vi "Parse (Write To EEPROM).vi"(7 "Message In":string) -> (8 "Word Sent To EEPROM":sgl)   [LabVIEW 2012, in "MicroStrain 3DM-GXx.lvlib"]
doc: "Parse the data from the 0xE4 message into the 16-bit word written to EEPROM."
uses:
  <instrlib>/MicroStrain 3DM-GXx/MicroStrain 3DM-GXx.lvlib
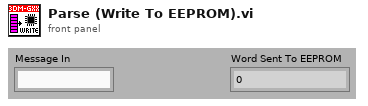
[diagram p1: front panel]
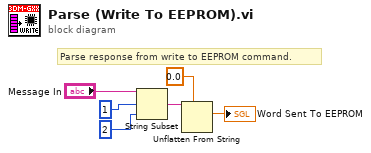
[diagram p0: block diagram]
diagram:
  # "Parse response from write to EEPROM command."
  n1 = String Subset(string="Message In", offset (0)=1, length (rest)=2 ("length (rest)")) -> (substring=w4:string)
  n2 = Unflatten From String(type=sgl 0.0, binary string=w4) -> (value=→"Word Sent To EEPROM":sgl)  [unwired: 3 in, 2 out]
